vi "Get AccessToken Instance.vi"(8 "error in (no error)":errorcluster, 11 "Oauth2 in":refnum<class "Oauth2.lvclass">) -> (0 "error out":errorcluster, 2 "OAuthAccessToken":refnum<class "OAuthAccessToken.lvclass">, 3 "Oauth2 out":refnum<class "Oauth2.lvclass">)   [LabVIEW 2013, in "Oauth2.lvclass"]
uses:
  Oauth2.lvclass
  OAuthToken/OAuthAccessToken.lvclass
  Oauth2.lvclass/Oauth2.ctl
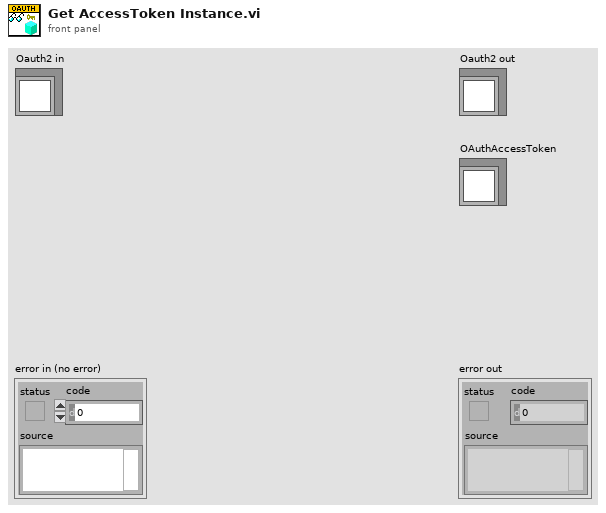
[diagram p1: front panel]
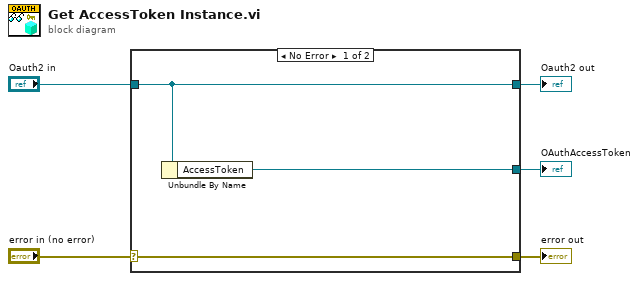
[diagram p0: block diagram]
diagram:
  n1 = case shown="No Error" "error in (no error)" {
    selector: "error in (no error)" -> [w8 w9]
    tunnel: [w8 w9] -> w4
    tunnel: [w7 w10] -> w2
    tunnel: "Oauth2 in" -> [w7 w10]
    tunnel: [w6 _] -> w1
    frame No Error {
      n2 = Unbundle By Name(w7) -> ("AccessToken"=w6:refnum<class "OAuthAccessToken.lvclass">)
    }
    frame Error {
    }
  }
  "error out" <- w4
  "Oauth2 out" <- w2
  "OAuthAccessToken" <- w1
